vi "Add Injector Shots (with separate stage section).vi"(8 "error in (no error)":errorcluster, 9 "Stage Names":string[](array[string]), 10 "# shots to add":u32, 11 "Injector Section Ref in":T1 format="%.0x") -> (0 "error out":errorcluster)   [LabVIEW 2019, in "Fuel Injector Analysis Addon System Explorer.lvlib"]
uses:
  Fuel Injector Analysis Addon System Explorer.lvlib
  <vilib>/NI VeriStand/Custom Device API/Custom Device Item Ref.ctl
  <vilib>/NI VeriStand/Custom Device API/Custom Device Channel.ctl
  <vilib>/NI VeriStand/Custom Device API/Custom Device Channel Type.ctl
  Addon Shared/Constants.vi
  <vilib>/NI VeriStand/Custom Device API/Custom Device API.lvlib
  Addon Shared/Fuel Injector Analysis Addon Shared.lvlib
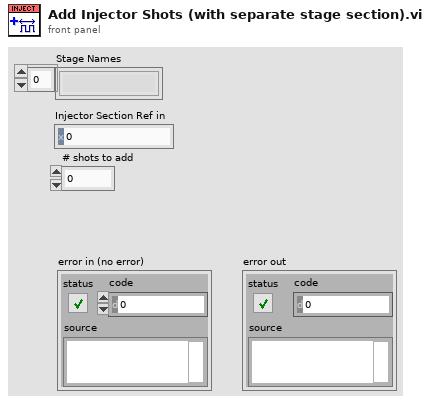
[diagram p1: front panel]
types:
  T1 = typedef "Custom Device API.lvlib/Custom Device Item Ref.ctl" = u64
  T2 = typedef "Custom Device API.lvlib/Custom Device Channel.ctl" = cluster{"Type":T3, "Units":string, "Default Value":dbl, "Faultable":bool, "Scalable":bool}
  T3 = typedef "Custom Device API.lvlib/Custom Device Channel Type.ctl" = enum16{"Input", "Output"}
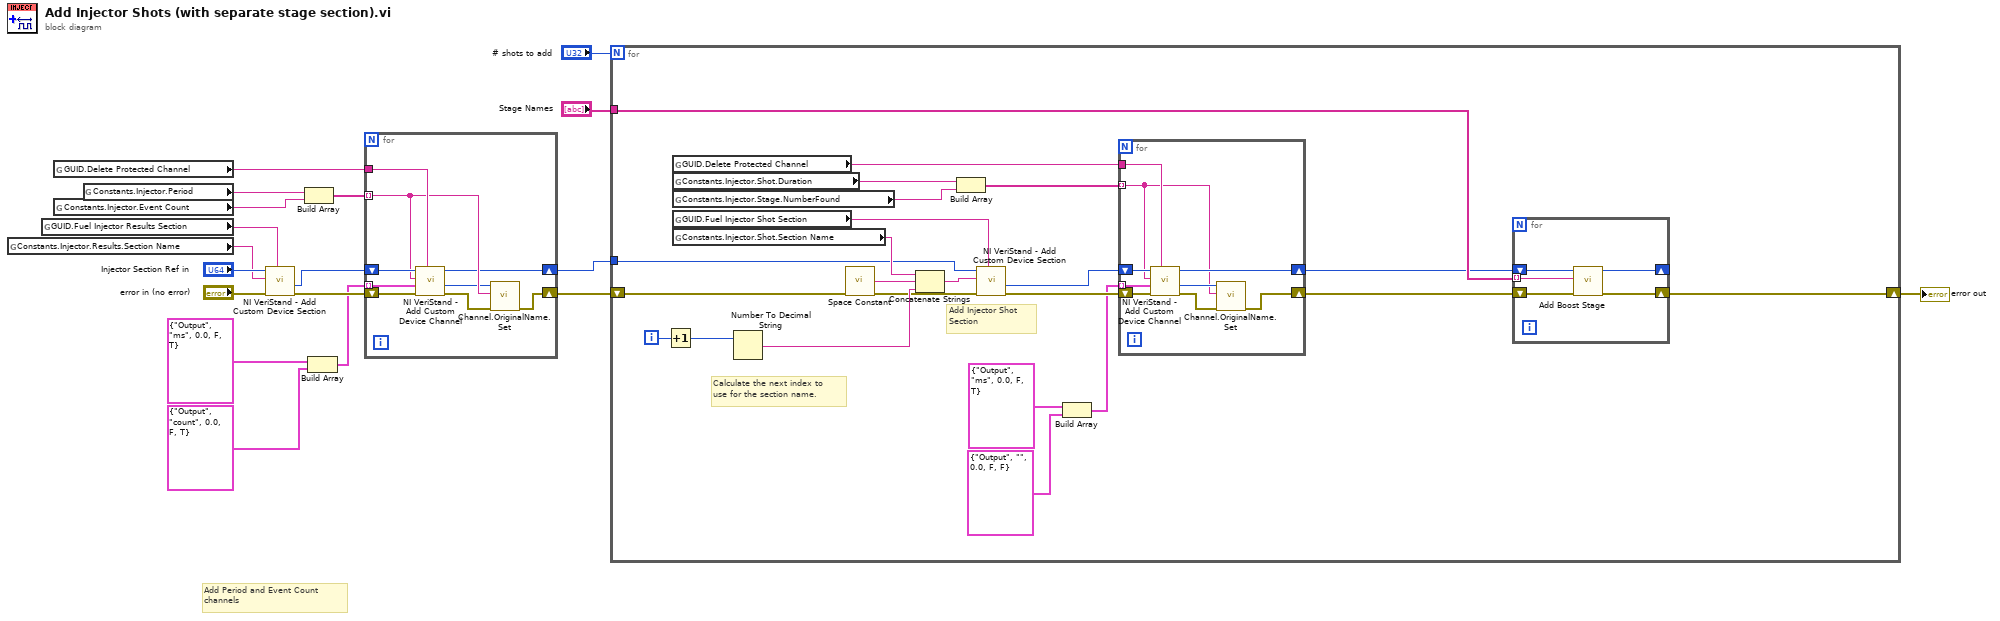
[diagram p0: block diagram]
diagram:
  # "Add Period and Event Count\nchannels"
  n1 = global read "Constants.vi" "Constants.Injector.Results.Section Name"() -> (w11:string)
  n2 = global read "Constants.vi" "GUID.Fuel Injector Results Section"() -> (w12:string)
  n3 = global read "Constants.vi" "GUID.Delete Protected Channel"() -> (w7:string)
  n4 = global read "Constants.vi" "Constants.Injector.Event Count"() -> (w6:string)
  n5 = global read "Constants.vi" "Constants.Injector.Period"() -> (w2:string)
  n6 = call <vilib>:"NI VeriStand - Add Custom Device Section.vi"("GUID (Default Section)"=w12, "error in (no error)"="error in (no error)", "Section Name"=w11, "Parent Ref in"="Injector Section Ref in") -> ("error out"=w16:errorcluster, "Section Ptr"=w15:T1)  [unwired: 4 in, 2 out]
  n7 = Build Array(w2, w6) -> (w3:string[])
  n8 = Build Array(T2 {"Type"=enum."Output", "Units"="ms", "Default Value"=0.0, "Faultable"=FALSE, "Scalable"=TRUE} ("Channel"), T2 {"Type"=enum."Output", "Units"="count", "Default Value"=0.0, "Faultable"=FALSE, "Scalable"=TRUE} ("Channel")) -> (w1:T2[])
  n9 = for {
    tunnel: w7 -> [w25]
    shift-right: [w23] -> w5
    shift-left: w16 -> [w27]
    shift-right: [w19] -> w4
    shift-left: w15 -> [w26]
    tunnel: w3 -> [w22] mode=indexing
    tunnel: w1 -> [w21] mode=indexing
    n10 = call <vilib>:"NI VeriStand - Add Custom Device Channel.vi"("GUID (Default Channel)"=w25, "error in (no error)"=w27, "Channel"=w21, "Channel Name"=w22, "Parent Ref in"=w26) -> ("error out"=w24:errorcluster, "Channel Ref"=w20:T1, "Parent Ref out"=w19:T1)  [unwired: 3 in, 1 out]
    n11 = call "Channel.OriginalName.Set.vi"("error in (no error)"=w24, "Constants.Channel Name"=w22, "Ref"=w20) -> ("error out"=w23:errorcluster)  [unwired: 7 in, 1 out]
  }
  n12 = for {
    N: "# shots to add" -> [_]
    tunnel: w4 -> [w42]
    shift-right: [w40] -> w18
    shift-left: w5 -> [w43]
    tunnel: "Stage Names" -> [w39]
    i -> [w48]
    # "Add Injector Shot\nSection"
    # "Calculate the next index to\nuse for the section name."
    n13 = Increment(x=w48) -> (x+1=w41:i32)
    n14 = global read "Constants.vi" "GUID.Delete Protected Channel"() -> (w37:string)
    n15 = global read "Constants.vi" "Constants.Injector.Shot.Duration"() -> (w33:string)
    n16 = global read "Constants.vi" "Constants.Injector.Stage.NumberFound"() -> (w32:string)
    n17 = global read "Constants.vi" "GUID.Fuel Injector Shot Section"() -> (w49:string)
    n18 = global read "Constants.vi" "Constants.Injector.Shot.Section Name"() -> (w47:string)
    n19 = Number To Decimal String(number=w41) -> (decimal integer string=w45:string)  [unwired: 1 in]
    n20 = call <vilib>:"Space Constant.vi"() -> ("String"=w46:string)
    n21 = Concatenate Strings(w47, w46, w45) -> (w44:string)
    n22 = Build Array(w33, w32) -> (w29:string[])
    n23 = call <vilib>:"NI VeriStand - Add Custom Device Section.vi"("GUID (Default Section)"=w49, "error in (no error)"=w43, "Section Name"=w44, "Parent Ref in"=w42) -> ("error out"=w30:errorcluster, "Section Ptr"=w31:T1)  [unwired: 4 in, 2 out]
    n24 = Build Array(T2 {"Type"=enum."Output", "Units"="ms", "Default Value"=0.0, "Faultable"=FALSE, "Scalable"=TRUE} ("Channel"), T2 {"Type"=enum."Output", "Units"="", "Default Value"=0.0, "Faultable"=FALSE, "Scalable"=FALSE} ("Channel")) -> (w28:T2[])
    n25 = for {
      tunnel: w37 -> [w57]
      shift-right: [w58] -> w38
      shift-left: w31 -> [w53]
      shift-right: [w54] -> w36
      shift-left: w30 -> [w52]
      tunnel: w29 -> [w51] mode=indexing
      tunnel: w28 -> [w50] mode=indexing
      n26 = call <vilib>:"NI VeriStand - Add Custom Device Channel.vi"("GUID (Default Channel)"=w57, "error in (no error)"=w52, "Channel"=w50, "Channel Name"=w51, "Parent Ref in"=w53) -> ("error out"=w55:errorcluster, "Channel Ref"=w56:T1, "Parent Ref out"=w58:T1)  [unwired: 3 in, 1 out]
      n27 = call "Channel.OriginalName.Set.vi"("error in (no error)"=w55, "Constants.Channel Name"=w51, "Ref"=w56) -> ("error out"=w54:errorcluster)  [unwired: 7 in, 1 out]
    }
    n28 = for {
      shift-right: [w63] -> w40
      shift-left: w36 -> [w62]
      shift-right: [w60] -> _
      shift-left: w38 -> [w61]
      tunnel: w39 -> [w59] mode=indexing
      n29 = call "Add Boost Stage.vi"("error in (no error)"=w62, "Stage Name"=w59, "Shot Section Item Ref"=w61) -> ("error out"=w63:errorcluster, "Shot Section Item Ref dup"=w60:T1)  [unwired: 7 in]
    }
  }
  "error out" <- w18
